vi "(SubVI)Chip ID Converter.vi"(11 "Chip ID":u8 format="%02x") -> (3 "Chip Type":string)   [LabVIEW 2020]
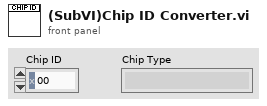
[diagram p1: front panel]
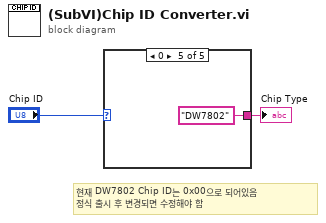
[diagram p0: block diagram]
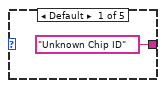
[diagram p2: hidden frame]
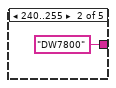
[diagram p3: hidden frame]
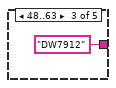
[diagram p4: hidden frame]
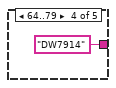
[diagram p5: hidden frame]
diagram:
  # "현재 DW7802 Chip ID는 0x00으로 되어있음\n정식 출시 후 변경되면 수정해야 함"
  n1 = case shown="0" "Chip ID" {
    tunnel: ["Unknown Chip ID" "DW7800" "DW7912" "DW7914" "DW7802"] -> w1
    frame Default {
    }
    frame 240..255 {
    }
    frame 48..63 {
    }
    frame 64..79 {
    }
    frame 0 {
    }
  }
  "Chip Type" <- w1
